vi "writeU64.vi"(8 "error in (no error)":errorcluster, 10 "Input":u64, 11 "M1M3SAL in":refnum<class "M1M3SAL.lvclass">) -> (0 "error out":errorcluster, 3 "M1M3SAL out":refnum<class "M1M3SAL.lvclass">)   [LabVIEW 2016, in "M1M3SupportCommunicator.lvlib" / "M1M3SAL.lvclass"]
uses:
  M1M3SAL.lvclass
  M1M3SAL.lvclass/M1M3SAL.ctl
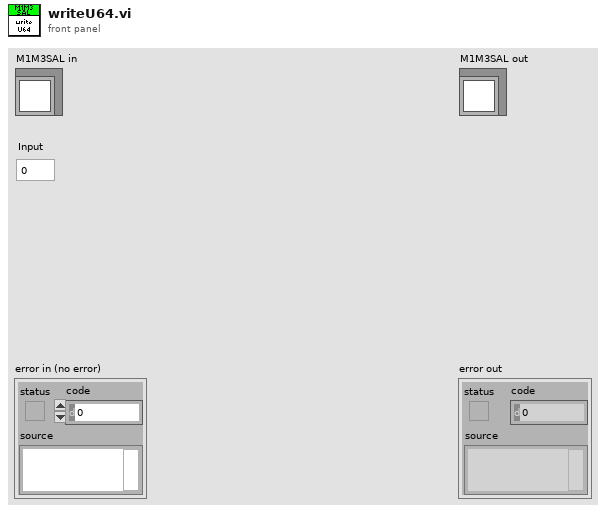
[diagram p1: front panel]
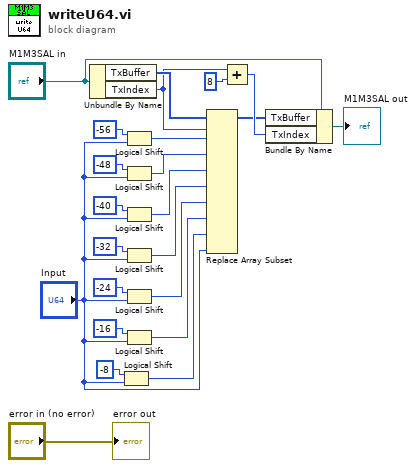
[diagram p0: block diagram]
diagram:
  n1 = Unbundle By Name("M1M3SAL in") -> ("TxBuffer"=w21:u8[], "TxIndex"=w20:i32)
  n2 = Logical Shift(y=i16 -8, x="Input") -> (x << y=w2:u64)
  n3 = Logical Shift(y=i16 -56, x="Input") -> (x << y=w8:u64)
  n4 = Logical Shift(y=i16 -48, x="Input") -> (x << y=w7:u64)
  n5 = Logical Shift(y=i16 -40, x="Input") -> (x << y=w6:u64)
  n6 = Logical Shift(y=i16 -32, x="Input") -> (x << y=w5:u64)
  n7 = Logical Shift(y=i16 -24, x="Input") -> (x << y=w4:u64)
  n8 = Logical Shift(y=i16 -16, x="Input") -> (x << y=w3:u64)
  n9 = Replace Array Subset(array=w21, new element #1=w8, index #1=w20, new element #2=w7, new element #3=w6, new element #4=w5, new element #5=w4, new element #6=w3, new element #7=w2, new element #8="Input") -> (w17:u8[])  [unwired: 7 in]
  n10 = Add(x=w20, y=8) -> (x+y=w18:i32)
  n11 = Bundle By Name(cluster="M1M3SAL in", "TxBuffer"=w17, "TxIndex"=w18) -> (→"M1M3SAL out":refnum<class "M1M3SAL.lvclass">)
  "error out" <- "error in (no error)"
